vi "setEvaluation.vi"(8 "error in (no error)":errorcluster, 10 "Evaluation":cluster{"F":dbl, "G":dbl, "H":dbl}, 11 "GraphNode in":refnum<class "GraphNode.lvclass">) -> (0 "error out":errorcluster, 3 "GraphNode out":refnum<class "GraphNode.lvclass">)   [LabVIEW 2013, in "GraphNode.lvclass"]
uses:
  GraphNode.lvclass
  GraphNode.lvclass/GraphNode.ctl
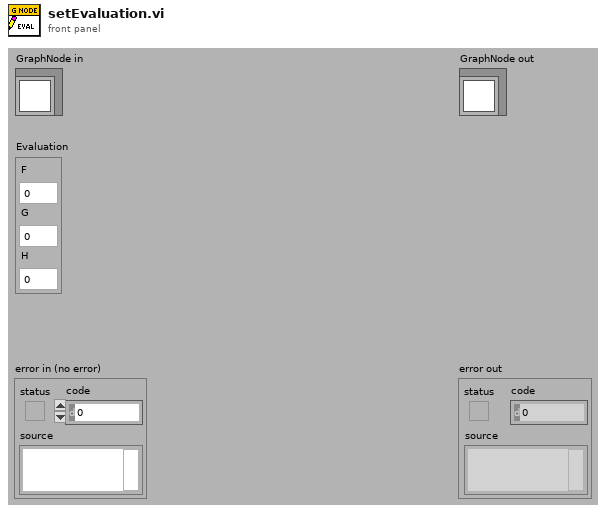
[diagram p1: front panel]
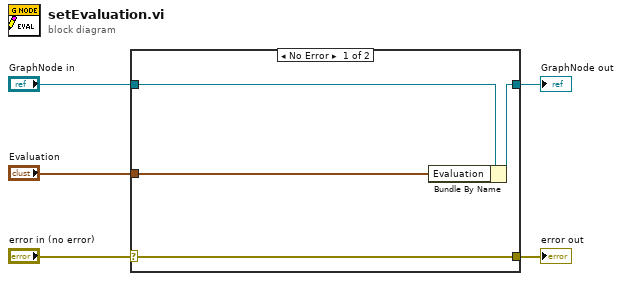
[diagram p0: block diagram]
diagram:
  n1 = case shown="No Error" "error in (no error)" {
    selector: "error in (no error)" -> [w9 w10]
    tunnel: [w9 w10] -> w4
    tunnel: [w7 w11] -> w2
    tunnel: "GraphNode in" -> [w8 w11]
    tunnel: "Evaluation" -> [w6 _]
    frame No Error {
      n2 = Bundle By Name(cluster=w8, "Evaluation"=w6) -> (w7:refnum<class "GraphNode.lvclass">)
    }
    frame Error {
    }
  }
  "error out" <- w4
  "GraphNode out" <- w2
